vi "MouliSOC.vi"(8 "errin":errorcluster caption="entrée d'erreur", 9 "SN":string, 10 "PN":string, 11 "chemin":path) -> (0 "errin 2":errorcluster caption="errin", 3 "Is30%?":bool)   [LabVIEW 2020]
uses:
  VG_SOC.vi
  OP400/VG/30%.vi
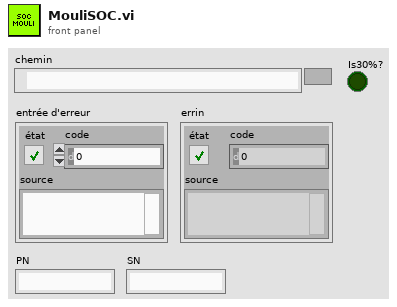
[diagram p1: front panel]
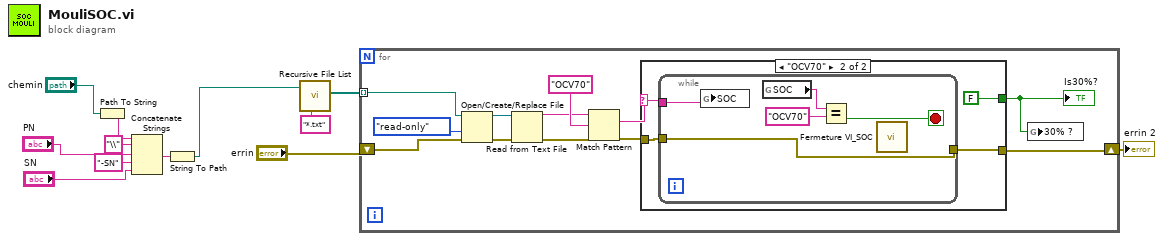
[diagram p0: block diagram]
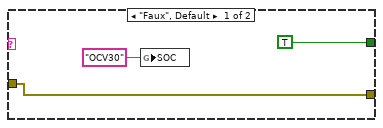
[diagram p2: hidden frame]
diagram:
  n1 = Path To String(path="chemin") -> (string=w2:string)
  n2 = Concatenate Strings(w2, "\\" ("chaîne"), "PN", "-SN" ("chaîne"), "SN") -> (w3:string)
  n3 = String To Path(string=w3) -> (path=w4:path)
  n4 = call <vilib>:"Recursive File List.vi"("pattern"="*.txt", "Folder Path"=w4) -> ("All Files in Dir"=w10:path[])  [unwired: 5 in, 4 out]
  n5 = for {
    shift-right: [w16] -> w9
    shift-left: "errin" -> [w23]
    tunnel: w10 -> [w21] mode=indexing
    n6 = Open/Create/Replace File(file path (use dialog)=w21, error in=w23, access (0:read/write)=enum16{"read/write", "read-only", "write-only"}."read-only" ("accès (0 : read/write)")) -> (refnum out=w18:refnum<file>, error out=w19:errorcluster)  [unwired: 3 in, 1 out]
    n7 = Read from Text File(file (use dialog)=w18, error in=w19) -> (text=w17:string, error out=w15:errorcluster)  [unwired: 2 in, 2 out]
    n8 = Match Pattern(string=w17, regular expression="OCV70" ("expression régulière")) -> (match substring=w14:string)  [unwired: 1 in, 3 out]
    n9 = case shown="\"OCV70\"" w14 {
      selector: w14 -> [_ w28]
      tunnel: [w26 w30] -> w16
      tunnel: w15 -> [w26 w29]
      tunnel: [TRUE FALSE] -> w13
      frame "Faux", Default {
        n10 = global write "VG_SOC.vi" "SOC"("OCV30" ("SOC")) -> ()
      }
      frame "OCV70" {
        n11 = while {
          tunnel: w28 -> [w35]
          tunnel: [w34] -> w30
          tunnel: w29 -> [w34]
          stop <- w31 stop-if-true
          n12 = global write "VG_SOC.vi" "SOC"(w35) -> ()
          n13 = global read "VG_SOC.vi" "SOC"() -> (w33:string)
          n14 = Equal?(x=w33, y="OCV70") -> (x = y?=w31:bool)
          n15 = call "Fermeture VI_SOC.vi"() -> ()  [unwired: 1 in]
        }
      }
    }
    "Is30%?" <- w13
    n16 = global write "30%.vi" "30% ?"(w13) -> ()
  }
  "errin 2" <- w9
